vi "ProdaNG.File.Write.vi"(5 "ProfInfo":string[](array[string]), 6 "Config":T1={"ShowUnreleased"=FALSE, "Param1"="", "ParamStartIdx"=0, "Slots"=1} {"Slots" min=1 max=2; "ParamStartIdx" min=0 max=1}, 7 "SlotNo":i32, 8 "error in (no error)":errorcluster, 9 "units":T2[](array[typedef]), 10 "Seq":T3, 11 "SeqFile Path":path) -> (0 "error out":errorcluster)   [LabVIEW 2016]
uses:
  ProdaNG.File.Sequence.ctl
  ProdaNG.Tree.Fglb.Value.ctl
  ProdaNG.File.Step.ctl
  Controls/ProdaNG.UnitSimple.ctl
  ProdaNG.Configurator.Config.ctl
  <vilib>/Utility/config.llb/Write Key (String).vi
  <vilib>/Utility/config.llb/Read Key (String).vi
  <vilib>/Utility/config.llb/NI_LVConfig.lvlib
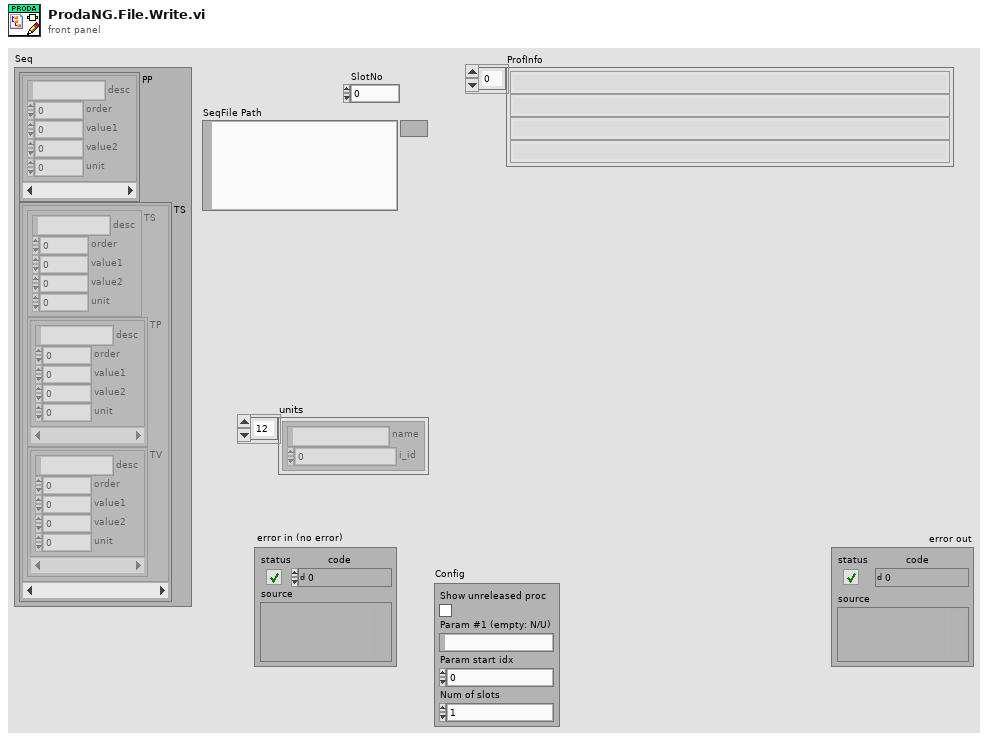
[diagram p1: front panel]
types:
  T1 = typedef "ProdaNG.Configurator.Config.ctl" = cluster{"ShowUnreleased":bool, "Param1":string, "ParamStartIdx":i32, "Slots":i32}
  T2 = typedef "ProdaNG.UnitSimple.ctl" = cluster{"name":string, "i_id":i32}
  T3 = typedef "ProdaNG.File.Sequence.ctl" = cluster{"PP":T4[], "TS":T5[]}
  T4 = typedef "ProdaNG.Tree.Fglb.Value.ctl" = cluster{"desc":string, "order":i32, "value1":dbl, "value2":dbl, "unit":i32}
  T5 = typedef "ProdaNG.File.Step.ctl" = cluster{"TS":T4, "TP":T4[], "TV":T4[]}
  T6 = typedef "NI_LVConfig.lvlib/Config Data RefNum.ctl" = refnum<k1>
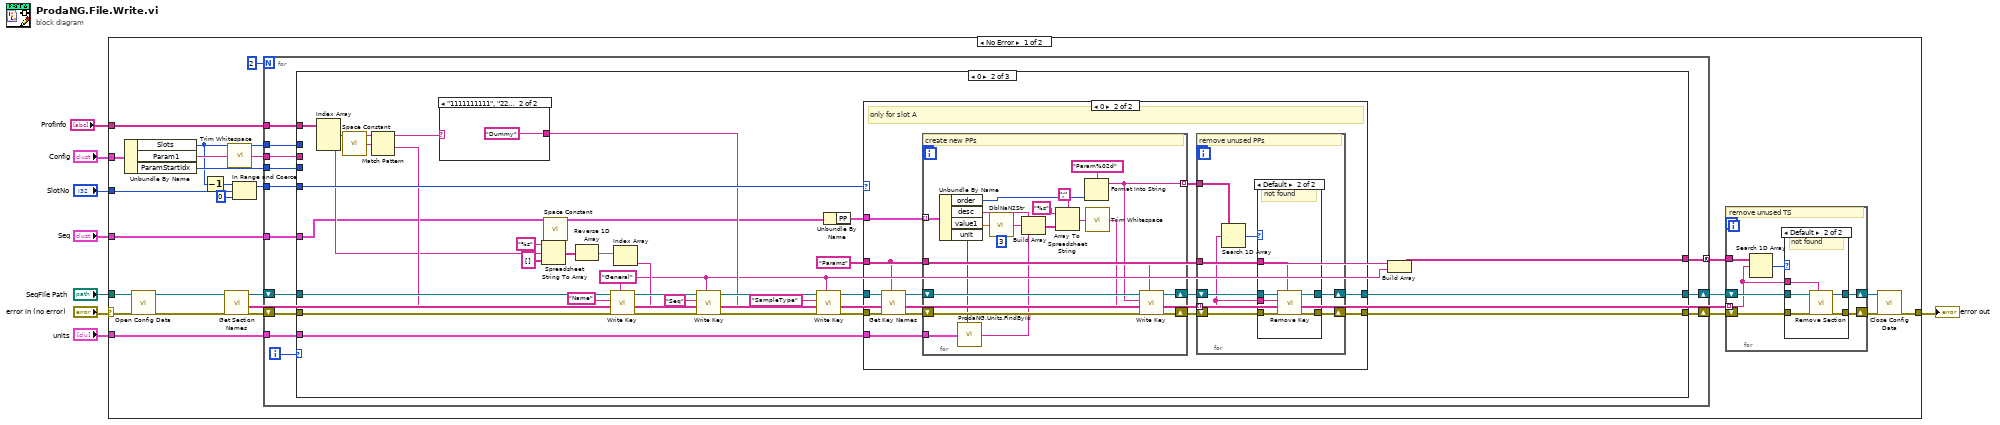
[diagram p0: block diagram]
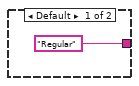
[diagram p3: hidden frame]
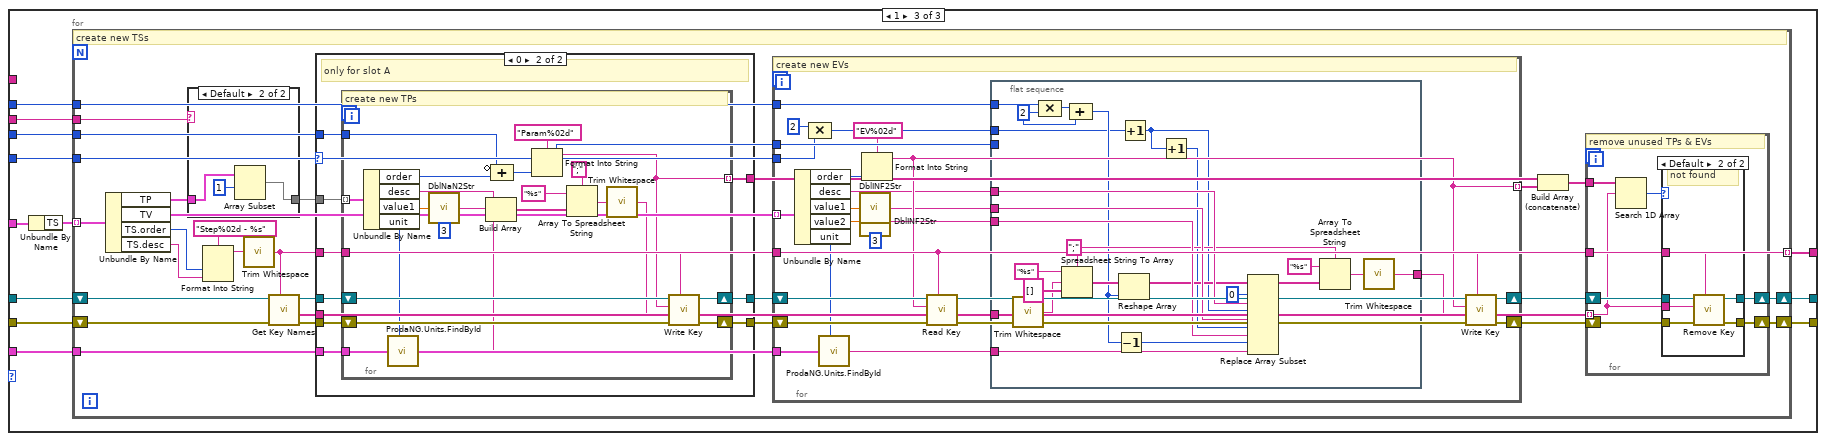
[diagram p6: hidden frame]
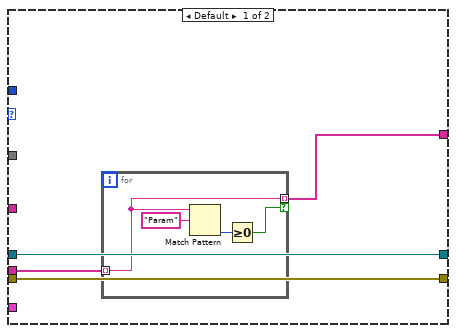
[diagram p8: hidden frame]
diagram:
  n1 = case shown="No Error" "error in (no error)" {
    selector: "error in (no error)" -> [w34 w300]
    tunnel: [w33 w300] -> w7
    tunnel: "SeqFile Path" -> [w32 _]
    tunnel: "units" -> [w24 _]
    tunnel: "SlotNo" -> [w31 _]
    tunnel: "Config" -> [w29 _]
    tunnel: "Seq" -> [w26 _]
    tunnel: "ProfInfo" -> [w23 _]
    frame No Error {
      n2 = Unbundle By Name(w29) -> ("Slots"=w11:i32, "Param1"=w30:string, "ParamStartIdx"=w27:i32)
      n3 = call <vilib>:"Open Config Data.vi"("error in (no error)"=w34, "configuration file path"=w32) -> ("error out"=w19:errorcluster, "refnum"=w20:T6)  [unwired: 7 in, 1 out]
      n4 = Decrement(x=w11) -> (x-1=w10:i32)
      n5 = call <vilib>:"Get Section Names.vi"("error in (no error)"=w19, "refnum"=w20) -> ("error out"=w22:errorcluster, "section names"=w13:string[], "refnum out"=w21:T6)  [unwired: 7 in]
      n6 = call <vilib>:"Trim Whitespace.vi"("string"=w30) -> ("trimmed string"=w28:string)  [unwired: 1 in]
      n7 = In Range and Coerce(upper limit=w10, x=w31, lower limit=0 ("y")) -> (coerced(x)=w12:i32)  [unwired: 1 out]
      n8 = for {
        N: 2 -> [_]
        tunnel: w12 -> [w45]
        tunnel: w28 -> [w44]
        tunnel: w27 -> [w43]
        tunnel: w26 -> [w42]
        shift-right: [w46] -> w17
        shift-left: w21 -> [w41]
        shift-right: [w47] -> w18
        shift-left: w22 -> [w40]
        tunnel: w24 -> [w38]
        tunnel: w23 -> [w37]
        tunnel: [w36] -> w14 mode=concatenating
        tunnel: w11 -> [w35]
        i -> [w39]
        n9 = case shown="0" w39 {
          tunnel: w40 -> [w48 w77 w142]
          tunnel: w41 -> [w49 w76 w141]
          tunnel: w45 -> [_ w82 w146]
          tunnel: [w48 w80 w140] -> w47
          tunnel: [w49 w79 w139] -> w46
          tunnel: w44 -> [_ _ w143]
          tunnel: w43 -> [_ _ w145]
          tunnel: w42 -> [_ w50 w148]
          tunnel: w38 -> [_ w78 w144]
          tunnel: w37 -> [_ w66 _]
          tunnel: [_ w51 w138] -> w36
          tunnel: w35 -> [_ _ w137]
          frame Default {
          }
          frame 0 {
            w52 = "General" ("regular expression")
            w53 = "Params" ("regular expression")
            n10 = Index Array(array=w66) -> (element #1=w65:string, element #3=w60:string)  [unwired: 3 in, 1 out]
            n11 = call <vilib>:"Space Constant.vi"() -> ("String"=w64:string)
            n12 = Match Pattern(string=w65, regular expression=w64) -> (before substring=w62:string, after substring=w63:string)  [unwired: 1 in, 2 out]
            n13 = case shown="\"1111111111\", \"2222222222\", \"3333333333\"" w62 {
              tunnel: ["Regular" ("key") "Dummy" ("key")] -> w61
              frame Default {
              }
              frame "1111111111", "2222222222", "3333333333" {
              }
            }
            n14 = call <vilib>:"Space Constant.vi"() -> ("String"=w57:string)
            n15 = Spreadsheet String To Array(delimiter (Tab)=w57, format string="%s", spreadsheet string=w60, array type (2D Dbl)=string[] []) -> (array=w56:string[])
            n16 = Reverse 1D Array(array=w56) -> (reversed array=w55:string[])
            n17 = call-poly <vilib>:"Write Key.vi"("section"=w52, "error in (no error)"=w77, "value"=w63, "key"="Name", "refnum"=w76) -> ("error out"=w69:errorcluster, "refnum out"=w74:T6)  [unwired: 4 in, 1 out]
            n18 = Index Array(array=w55) -> (element=w54:string)  [unwired: 1 in]
            n19 = call-poly <vilib>:"Write Key.vi"("section"=w52, "error in (no error)"=w69, "value"=w54, "key"="Seq", "refnum"=w74) -> ("error out"=w70:errorcluster, "refnum out"=w73:T6)  [unwired: 4 in, 1 out]
            n20 = call-poly <vilib>:"Write Key.vi"("section"=w52, "error in (no error)"=w70, "value"=w61, "key"="SampleType", "refnum"=w73) -> ("error out"=w71:errorcluster, "refnum out"=w72:T6)  [unwired: 4 in, 1 out]
            n21 = Unbundle By Name(w50) -> ("PP"=w81:T4[])
            n22 = case shown="0" w82 {
              tunnel: w71 -> [w86 w98]
              tunnel: w72 -> [w85 w96]
              tunnel: [w85 w92] -> w79
              tunnel: [w86 w91] -> w80
              tunnel: w81 -> [_ w99]
              tunnel: w53 -> [_ w88]
              tunnel: w78 -> [_ w87]
              frame Default {
              }
              frame 0 {
                # "only for slot A"
                n23 = call <vilib>:"Get Key Names.vi"("section"=w88, "error in (no error)"=w98, "refnum"=w96) -> ("error out"=w97:errorcluster, "key names"=w89:string[], "refnum out"=w95:T6)  [unwired: 5 in, 1 out]
                n24 = for {
                  shift-right: [w117] -> w94
                  shift-left: w95 -> [w119]
                  shift-right: [w116] -> w93
                  shift-left: w97 -> [w118]
                  tunnel: w99 -> [w115] mode=indexing
                  tunnel: w88 -> [w105]
                  tunnel: [w104] -> w90 mode=indexing
                  tunnel: w87 -> [w103]
                  # "create new PPs"
                  n25 = Unbundle By Name(w115) -> ("order"=w100:i32, "desc"=w111:string, "value1"=w114:dbl, "unit"=w102:i32)
                  n26 = call "ProdaNG.Units.FindById.vi"("units"=w103, "unit id"=w102) -> ("unit str"=w101:string)  [unwired: 1 in]
                  n27 = call "DblNaN2Str.vi"("Numeric"=w114, "precision (6)"=i16 3) -> ("string"=w112:string)
                  n28 = Build Array(w111, w112, w101) -> (w110:string[])
                  n29 = Array To Spreadsheet String(delimiter (Tab)=";", array=w110, 3:"%s" ("format string")) -> (spreadsheet string=w106:string)
                  n30 = Format Into String(format string="Param%02d", w100) -> (resulting string=w104:string)  [unwired: 2 in, 1 out]
                  n31 = call <vilib>:"Trim Whitespace.vi"("string"=w106) -> ("trimmed string"=w107:string)  [unwired: 1 in]
                  n32 = call-poly <vilib>:"Write Key.vi"("section"=w105, "error in (no error)"=w118, "value"=w107, "key"=w104, "refnum"=w119) -> ("error out"=w116:errorcluster, "refnum out"=w117:T6)  [unwired: 4 in, 1 out]
                }
                n33 = for {
                  tunnel: w89 -> [w121] mode=indexing
                  shift-right: [w128] -> w91
                  shift-left: w93 -> [w125]
                  shift-right: [w127] -> w92
                  shift-left: w94 -> [w126]
                  tunnel: w90 -> [w124]
                  tunnel: w88 -> [w122]
                  # "remove unused PPs"
                  n34 = Search 1D Array(1D array=w124, element=w121) -> (index of element=w123:i32)  [unwired: 1 in]
                  n35 = case shown="Default" w123 {
                    tunnel: [w129 w136] -> w128
                    tunnel: [w130 w135] -> w127
                    tunnel: w126 -> [w130 w134]
                    tunnel: w125 -> [w129 w133]
                    tunnel: w122 -> [_ w132]
                    tunnel: w121 -> [_ w131]
                    frame 0.. {
                    }
                    frame Default {
                      # "not found"
                      n36 = call <vilib>:"Remove Key.vi"("section"=w132, "error in (no error)"=w133, "key"=w131, "refnum"=w134) -> ("error out"=w136:errorcluster, "refnum out"=w135:T6)  [unwired: 5 in, 1 out]
                    }
                  }
                }
              }
            }
            n37 = Build Array(w53, w52) -> (w51:string[])
          }
          frame 1 {
            n38 = Unbundle By Name(w148) -> ("TS"=w147:T5[])
            n39 = for {
              tunnel: w147 -> [w174] mode=indexing
              shift-right: [w166] -> w139
              shift-left: w141 -> [w170]
              shift-right: [w165] -> w140
              shift-left: w142 -> [w171]
              tunnel: w146 -> [w149]
              tunnel: w145 -> [w167]
              tunnel: [w155] -> w138 mode=indexing
              tunnel: w144 -> [w154]
              tunnel: w143 -> [w153]
              tunnel: w137 -> [w150]
              # "create new TSs"
              n40 = Unbundle By Name(w174) -> ("TP"=w152:T4[], "TV"=w164:T4[], "TS.order"=w168:i32, "TS.desc"=w169:string)
              n41 = case shown="Default" w153 {
                tunnel: w152 -> [w175 w178]
                tunnel: [w175 w177] -> w151
                frame "" {
                }
                frame Default {
                  n42 = Array Subset(array=w178, index=1) -> (w177:T4[])  [unwired: 1 in]
                }
              }
              n43 = Format Into String(format string="Step%02d - %s", w168, w169) -> (resulting string=w172:string)  [unwired: 2 in, 1 out]
              n44 = call <vilib>:"Trim Whitespace.vi"("string"=w172) -> ("trimmed string"=w155:string)  [unwired: 1 in]
              n45 = call <vilib>:"Get Key Names.vi"("section"=w155, "error in (no error)"=w171, "refnum"=w170) -> ("error out"=w163:errorcluster, "key names"=w156:string[], "refnum out"=w162:T6)  [unwired: 5 in, 1 out]
              n46 = case shown="0" w149 {
                tunnel: w151 -> [_ w195]
                tunnel: w155 -> [_ w194]
                tunnel: w167 -> [_ w193]
                tunnel: w163 -> [w181 w192]
                tunnel: w162 -> [w182 w191]
                tunnel: [w179 w190] -> w161
                tunnel: [w182 w189] -> w160
                tunnel: [w181 w188] -> w159
                tunnel: w156 -> [w180 _]
                tunnel: w154 -> [_ w187]
                frame Default {
                  n47 = for {
                    tunnel: w180 -> [w185] mode=indexing
                    tunnel: [w185] -> w179 mode=indexing if=w183
                    n48 = Match Pattern(string=w185, regular expression="Param") -> (offset past match=w184:i32)  [unwired: 1 in, 3 out]
                    n49 = Greater Or Equal To 0?(x=w184) -> (x >= 0?=w183:bool)
                  }
                }
                frame 0 {
                  # "only for slot A"
                  n50 = for {
                    shift-right: [w215] -> w189
                    shift-left: w191 -> [w217]
                    shift-right: [w214] -> w188
                    shift-left: w192 -> [w216]
                    tunnel: w193 -> [w212]
                    tunnel: w195 -> [w211] mode=indexing
                    tunnel: w194 -> [w200]
                    tunnel: [w199] -> w190 mode=indexing
                    tunnel: w187 -> [w196]
                    # "create new TPs"
                    n51 = Unbundle By Name(w211) -> ("order"=w210:i32, "desc"=w206:string, "value1"=w209:dbl, "unit"=w198:i32)
                    n52 = call "ProdaNG.Units.FindById.vi"("units"=w196, "unit id"=w198) -> ("unit str"=w197:string)  [unwired: 1 in]
                    n53 = call "DblNaN2Str.vi"("Numeric"=w209, "precision (6)"=i16 3) -> ("string"=w207:string)
                    n54 = Build Array(w206, w207, w197) -> (w205:string[])
                    n55 = Compound Arithmetic op=ADD(invert w212, w210) -> (w213:i32)
                    n56 = Format Into String(format string="Param%02d", w213) -> (resulting string=w199:string)  [unwired: 2 in, 1 out]
                    n57 = Array To Spreadsheet String(delimiter (Tab)=";", array=w205, 3:"%s" ("format string")) -> (spreadsheet string=w201:string)
                    n58 = call <vilib>:"Trim Whitespace.vi"("string"=w201) -> ("trimmed string"=w202:string)  [unwired: 1 in]
                    n59 = call-poly <vilib>:"Write Key.vi"("section"=w200, "error in (no error)"=w216, "value"=w202, "key"=w199, "refnum"=w217) -> ("error out"=w214:errorcluster, "refnum out"=w215:T6)  [unwired: 4 in, 1 out]
                  }
                }
              }
              n60 = for {
                shift-right: [w245] -> _
                shift-left: w160 -> [w236]
                shift-right: [w244] -> _
                shift-left: w159 -> [w237]
                tunnel: w164 -> [w239] mode=indexing
                tunnel: w155 -> [w233]
                tunnel: [w231] -> w157 mode=indexing
                tunnel: w149 -> [w238]
                tunnel: w154 -> [w223]
                tunnel: w150 -> [w222]
                tunnel: w149 -> [w221]
                w227 = i16 3 ("precision (6)")
                # "create new EVs"
                n61 = Unbundle By Name(w239) -> ("order"=w240:i32, "desc"=w229:string, "value1"=w243:dbl, "value2"=w241:dbl, "unit"=w225:i32)
                n62 = Compound Arithmetic op=MULTIPLY(2 ("value"), w221) -> (w219:i32)
                n63 = call "ProdaNG.Units.FindById.vi"("units"=w223, "unit id"=w225) -> ("unit str"=w224:string)  [unwired: 1 in]
                n64 = call "DblINF2Str.vi"("Numeric"=w243, "precision (6)"=w227) -> ("string"=w228:string)
                n65 = call "DblINF2Str.vi"("Numeric"=w241, "precision (6)"=w227) -> ("string"=w226:string)
                n66 = Format Into String(format string="EV%02d", w240) -> (resulting string=w231:string)  [unwired: 2 in, 1 out]
                n67 = call-poly <vilib>:"Read Key.vi"("section"=w233, "error in (no error)"=w237, "key"=w231, "refnum"=w236) -> ("error out"=w234:errorcluster, "value"=w230:string, "refnum out"=w235:T6)  [unwired: 4 in, 1 out]
                n68 = flat-sequence {
                  tunnel: [w268] -> w242
                  tunnel: w238 -> [_]
                  tunnel: w230 -> [w266]
                  tunnel: w229 -> [w265]
                  tunnel: w228 -> [w264]
                  tunnel: w226 -> [w263]
                  tunnel: w224 -> [w256]
                  tunnel: w222 -> [w254]
                  tunnel: w219 -> [w249]
                  frame #0 {
                    w250 = 2 ("value")
                    w257 = ";" ("delimiter (Tab)")
                    n69 = call <vilib>:"Trim Whitespace.vi"("string"=w266) -> ("trimmed string"=w260:string)  [unwired: 1 in]
                    n70 = Compound Arithmetic op=MULTIPLY(w254, w250) -> (w253:i32)
                    n71 = Spreadsheet String To Array(delimiter (Tab)=w257, format string="%s", spreadsheet string=w260, array type (2D Dbl)=string[] []) -> (array=w259:string[])
                    n72 = Compound Arithmetic op=unknown(w253, w250) -> (w252:i32)
                    n73 = Decrement(x=w252) -> (x-1=w251:i32)
                    n74 = Reshape Array(w259, w252) -> (w255:string[])
                    n75 = Increment(x=w249) -> (x+1=w247:i32)
                    n76 = Increment(x=w247) -> (x+1=w246:i32)
                    n77 = Replace Array Subset(array=w255, new element #1=w265, index #1=0 ("index"), new element #2=w264, index #2=w247, new element #3=w263, index #3=w246, new element #4=w256, index #4=w251) -> (w258:string[])
                    n78 = Array To Spreadsheet String(delimiter (Tab)=w257, array=w258, 3:"%s" ("format string")) -> (spreadsheet string=w267:string)
                    n79 = call <vilib>:"Trim Whitespace.vi"("string"=w267) -> ("trimmed string"=w268:string)  [unwired: 1 in]
                  }
                }
                n80 = call-poly <vilib>:"Write Key.vi"("section"=w233, "error in (no error)"=w234, "value"=w242, "key"=w231, "refnum"=w235) -> ("error out"=w244:errorcluster, "refnum out"=w245:T6)  [unwired: 4 in, 1 out]
              }
              n81 = Build Array (concatenate)(w161, w157) -> (w158:string[])
              n82 = for {
                tunnel: w156 -> [w271] mode=indexing
                shift-right: [w277] -> w165
                shift-left: w159 -> [w274]
                shift-right: [w276] -> w166
                shift-left: w160 -> [w275]
                tunnel: w158 -> [w273]
                tunnel: w155 -> [w270]
                # "remove unused TPs & EVs"
                n83 = Search 1D Array(1D array=w273, element=w271) -> (index of element=w272:i32)  [unwired: 1 in]
                n84 = case shown="Default" w272 {
                  tunnel: [w278 w285] -> w277
                  tunnel: [w279 w284] -> w276
                  tunnel: w275 -> [w279 w283]
                  tunnel: w274 -> [w278 w282]
                  tunnel: w271 -> [_ w281]
                  tunnel: w270 -> [_ w280]
                  frame 0.. {
                  }
                  frame Default {
                    # "not found"
                    n85 = call <vilib>:"Remove Key.vi"("section"=w280, "error in (no error)"=w282, "key"=w281, "refnum"=w283) -> ("error out"=w285:errorcluster, "refnum out"=w284:T6)  [unwired: 5 in, 1 out]
                  }
                }
              }
            }
          }
        }
      }
      n86 = for {
        tunnel: w13 -> [w286] mode=indexing
        shift-right: [w292] -> w15
        shift-left: w18 -> [w289]
        shift-right: [w291] -> w16
        shift-left: w17 -> [w290]
        tunnel: w14 -> [w288]
        # "remove unused TS"
        n87 = Search 1D Array(1D array=w288, element=w286) -> (index of element=w287:i32)  [unwired: 1 in]
        n88 = case shown="Default" w287 {
          tunnel: [w293 w299] -> w292
          tunnel: [w294 w298] -> w291
          tunnel: w290 -> [w294 w297]
          tunnel: w289 -> [w293 w296]
          tunnel: w286 -> [_ w295]
          frame 0.. {
          }
          frame Default {
            # "not found"
            n89 = call <vilib>:"Remove Section.vi"("section"=w295, "error in (no error)"=w296, "refnum"=w297) -> ("error out"=w299:errorcluster, "refnum out"=w298:T6)  [unwired: 6 in, 1 out]
          }
        }
      }
      n90 = call <vilib>:"Close Config Data.vi"("error in (no error)"=w15, "refnum"=w16) -> ("error out"=w33:errorcluster)  [unwired: 8 in, 1 out]
    }
    frame Error {
    }
  }
  "error out" <- w7
